vi "Tx Stream Controller (FPGA).vi"() -> ()   [LabVIEW 2016]
doc: "Controls the generation and reception of data transferred from the Host to the FPGA.\nPort 0 receives data from the Port 0 TX Input DMA FIFO and transmits that data to Port 1.\nPort 1 receives data from the Port 1 TX Input DMA FIFO and transmits that data to Port 0."
uses:
  <instrlib>/_niInstr/Streaming/v1/Common/Stream State.ctl
  <vilib>/Platform/TimedLoop/XDataNode/timing_clust.ctl
  <vilib>/Platform/TimedLoop/XDataNode/nitl_modes.ctl
  <vilib>/Platform/TimedLoop/XDataNode/wakeup.ctl
  <instrlib>/_niInstr/CLIP Adapters/v1/FPGA/AXI4-Lite/FXP32 Address - FXP32 Data/Public/CLIP Resources.ctl
  <instrlib>/_niInstr/CLIP Adapters/v1/FPGA/AXI4-Lite/Address Space Collection/niInstr AXI4-Lite Address Space Collection v1 FPGA.lvclass
  C:/Program Files (x86)/National Instruments/LabVIEW 2016/instr.lib/_niInstr/Instruction Framework/v1/FPGA/Interfaces/Address Space Collection/Address Space Collection.lvclass
  <instrlib>/_niInstr/FIFO Register Bus/v1/FPGA/niInstr FIFO Register Bus v1 FPGA.lvclass
  C:/Program Files (x86)/National Instruments/LabVIEW 2016/instr.lib/_niInstr/Instruction Framework/v1/FPGA/Interfaces/Instruction Producer/Instruction Producer.lvclass
  <instrlib>/_niInstr/CLIP Adapters/v1/FPGA/AXI4-Stream/Reader FXP64x1/niInstr AXI4-Stream Reader FXP64x1 v1 FPGA.lvclass
  C:/Program Files (x86)/National Instruments/LabVIEW 2016/instr.lib/_niInstr/CLIP Adapters/v1/FPGA/AXI4-Stream/Reader/niInstr AXI4-Stream Reader v1 FPGA.lvclass
  <instrlib>/_niInstr/CLIP Adapters/v1/FPGA/AXI4-Stream/Writer FXP64x1/niInstr AXI4-Stream Writer FXP64x1 v1 FPGA.lvclass
  C:/Program Files (x86)/National Instruments/LabVIEW 2016/instr.lib/_niInstr/CLIP Adapters/v1/FPGA/AXI4-Stream/Writer/niInstr AXI4-Stream Writer v1 FPGA.lvclass
  <vilib>/rvi/Emulation/niFpgaSctlEmulationGetInTimedLoop.vi
  <vilib>/rvi/Emulation/niFpgaEmulationReportErrorSimple.vi
  <vilib>/rvi/Emulation/niFpgaGetClockAttributes.vi
  <vilib>/rvi/Emulation/niFpgaCriticalErrorInLSC.vi
  <instrlib>/_niInstr/Basic Elements/v1/FPGA/Private/Read U64 FIFO.vi
  <instrlib>/_niInstr/Basic Elements/v1/FPGA/Private/Write U64 FIFO.vi
  <vilib>/rvi/Emulation/niFpgaProcessEmulError.vi
  <vilib>/rvi/eio/common/nirviEmuTemplateMethod_errors.vi
  <vilib>/Platform/TimedLoop/XDataNode/XDataNode.xnode
  <vilib>/eio/EIONode/EIONode.xnode
  <vilib>/Platform/TimedLoop/XDataNode/XDNodeRunTimeDep.lvlib
  <instrlib>/_niInstr/CLIP Adapters/v1/FPGA/AXI4-Stream/Writer/niInstr AXI4-Stream Writer v1 FPGA.lvclass
  <instrlib>/_niInstr/CLIP Adapters/v1/FPGA/AXI4-Stream/Reader/niInstr AXI4-Stream Reader v1 FPGA.lvclass
  <instrlib>/_niInstr/Basic Elements/v1/FPGA/niInstr Basic Elements v1 FPGA.lvlib
  SubVIS/Aurora Stream (NI 6592R) (FPGA).lvlib
  <instrlib>/_niInstr/Streaming/v1/FPGA/niInstr Streaming v1 FPGA.lvlib
  <instrlib>/_niInstr/Streaming/v1/Common/niInstr Streaming v1 Common.lvlib
  <instrlib>/_niInstr/Instruction Framework/v1/FPGA/Top Level Bus/Register Configuration/Register Configuration.lvclass
  <instrlib>/_niInstr/CLIP Adapters/v1/FPGA/AXI4-Lite/FXP32 Address - FXP32 Data/niInstr AXI4-Lite - FXP32 Address - FXP32 Data v1 FPGA.lvclass
panel:
  out "Er.Port 3":u32
  out "Er.Port 2":u32
  out "Er.Port 1":u32
  out "Er.Port 0":u32
  in  "Simulated data":bool
  in  "Reset":bool
  out "Port 3 Link Reset":bool
  out "Port 1 Link Reset":bool
  in  "Port 3 PMA Init":bool
  in  "Port 1 PMA Init":bool
  out "fifo reg bus data 0":u64
  out "fifo reg bus status 0":u32
  in  "fifo reg bus ctrl 0":u32
  in  "Port 0 PMA Init":bool
  in  "Port 2 PMA Init":bool
  out "Port 0 Debug Info":T1
  out "Port 0 Link Reset":bool
  out "Port 2 Link Reset":bool
  out "sFrontEndConfig_Complete":bool
  out "Port 2 Debug Info":T1
  out "stream.state 5":T2
  out "stream.samples transferred 5":u64
  out "stream.metadata 5":u64
  in  "stream.num samples 5":u64
  in  "stream.request state 5":T2
  out "stream.state 4":T2
  out "stream.samples transferred 4":u64
  out "stream.metadata 4":u64
  in  "stream.num samples 4":u64
  in  "stream.request state 4":T2
  in  "stream.request state 0":T2
  in  "stream.num samples 0":u64
  out "stream.metadata 0":u64
  out "stream.samples transferred 0":u64
  out "stream.state 0":T2
  in  "stream.num samples 1":u64
  in  "stream.request state 1":T2
  out "stream.state 1":T2
  out "stream.samples transferred 1":u64
  out "stream.metadata 1":u64
  in  "stream.request state 6":T2
  in  "stream.num samples 6":u64
  out "stream.metadata 6":u64
  out "stream.samples transferred 6":u64
  out "stream.state 6":T2
  in  "stream.request state 7":T2
  in  "stream.num samples 7":u64
  out "stream.metadata 7":u64
  out "stream.samples transferred 7":u64
  out "stream.state 7":T2
  out "Port 3 Debug Info":T1
  in  "stream.request state 2":T2
  in  "stream.num samples 2":u64
  out "stream.metadata 2":u64
  out "stream.samples transferred 2":u64
  out "stream.state 2":T2
  in  "stream.request state 3":T2
  in  "stream.num samples 3":u64
  out "stream.metadata 3":u64
  out "stream.samples transferred 3":u64
  out "stream.state 3":T2
  out "Port 1 Debug Info":T1
  # "Port 0"
  # "Port 2"
  # "Port 1"
  # "Port 3"
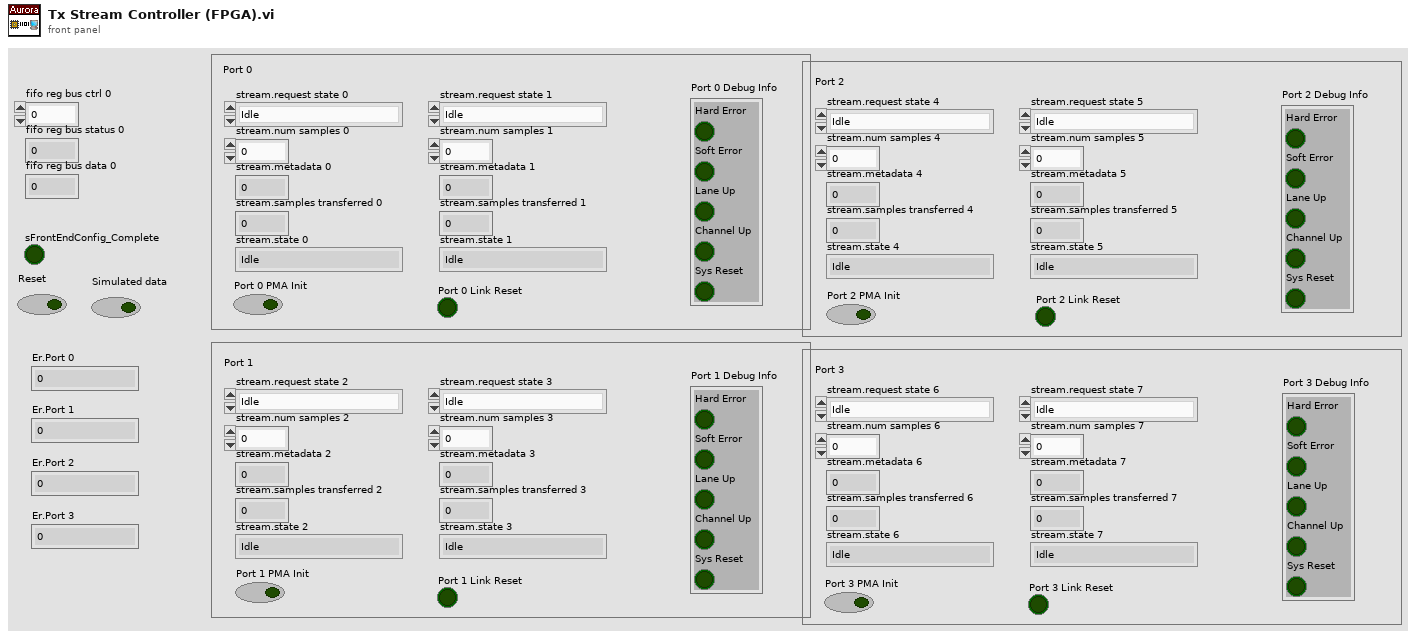
[diagram p1: front panel]
types:
  T1 = cluster{"Hard Error":bool, "Soft Error":bool, "Lane Up":bool, "Channel Up":bool, "Sys Reset":bool}
  T2 = typedef "niInstr Streaming v1 Common.lvlib/Stream State.ctl" = enum8{"Idle", "Finite Transfer", "Continuous", "Done", "Error", "Not Ready", "Cancel"}
  T3 = cluster{"Hard Error":refnum<k21>, "Soft Error":refnum<k21>, "Lane Up":refnum<k21>, "Channel Up":refnum<k21>, "Sys Reset":refnum<k21>}
  T4 = cluster{"m_axis_tvalid":refnum<k21>, "m_axis_tdata":refnum<k21>}
  T5 = cluster{"s_axis_tvalid":refnum<k21>, "s_axis_tdata":refnum<k21>, "s_axis_tready":refnum<k21>}
  T6 = typedef "niInstr AXI4-Lite - FXP32 Address - FXP32 Data v1 FPGA.lvclass/CLIP Resources.ctl" = cluster{"s_axi_araddr":refnum<k21>, "s_axi_arvalid":refnum<k21>, "s_axi_arready":refnum<k21>, "s_axi_rdata":refnum<k21>, "s_axi_rresp":refnum<k21>, "s_axi_rvalid":refnum<k21>, "s_axi_rready":refnum<k21>, "s_axi_awaddr":refnum<k21>, "s_axi_awvalid":refnum<k21>, "s_axi_awready":refnum<k21>, "s_axi_wdata":refnum<k21>, "s_axi_wstrb":refnum<k21>, "s_axi_wvalid":refnum<k21>, "s_axi_wready":refnum<k21>, "s_axi_bresp":refnum<k21>, "s_axi_bvalid":refnum<k21>, "s_axi_bready":refnum<k21>}
  T7 = typedef "XDNodeRunTimeDep.lvlib/timing_clust.ctl" = cluster{"Expected End [f-1]":u64, "Actual End [f-1]":u64, "Finished Late? [f-1]":bool, "Expected End [i-1]":u64, "Actual End [i-1]":u64, "Finished Late? [i-1]":bool, "Expected Start [i]":u64, "Actual Start [i]":u64, "Expected Start [f]":u64, "Actual Start [f]":u64, "Source Name":string, "Structure Name":string, "Period":i64, "Deadline":i64, "Offset":i64, "Start":i64, "Priority":i32, "Timeout":i32, "Mode":T8, "Wakeup Reason":T9, "Error":errorcluster, "Source Type":string, "Secondary Source Type":string, "Global End Time":u64, "Global Start Time":u64, "Frame Duration":u64, "Iteration Duration":u64, "Assigned CPU":i32, "I/O Scan Engine Mode":u32}
  T8 = typedef "XDNodeRunTimeDep.lvlib/nitl_modes.ctl" = enum32{"No Change", "Process missed periods, maintain original phase", "Discard missed periods, maintain original phase", "Process missed periods, ignore original phase", "Discard missed periods, ignore original phase"}
  T9 = typedef "XDNodeRunTimeDep.lvlib/wakeup.ctl" = enum32{"Normal", "Aborted", "Asynchronous wakeup", "Timing source error", "Timed loop error", "Timeout"}
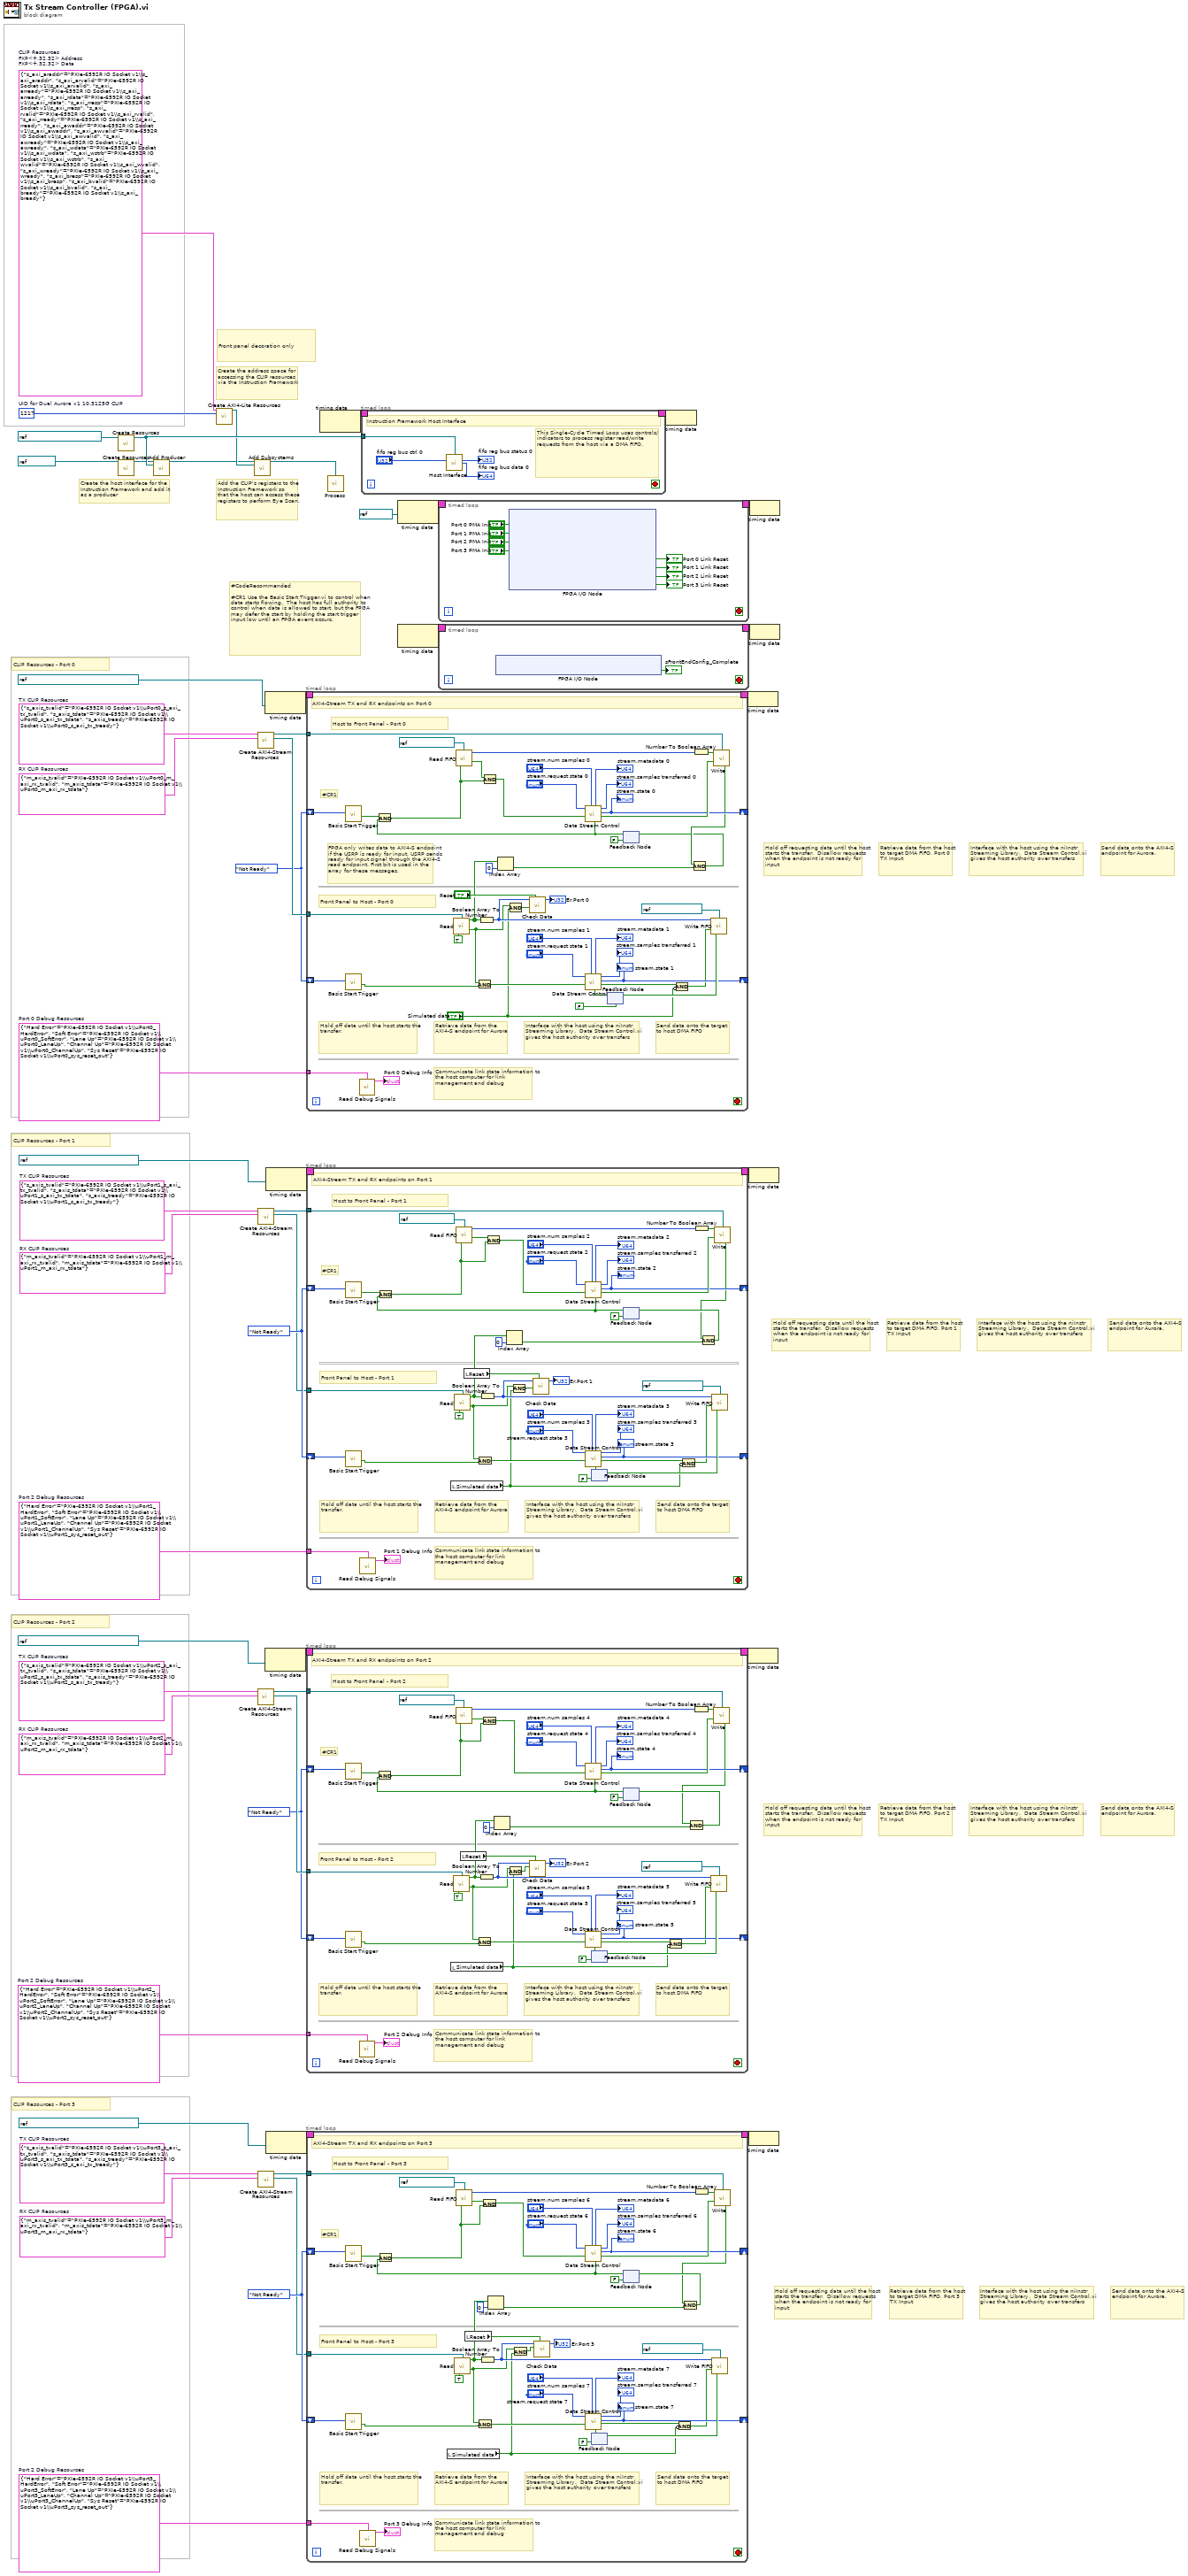
[diagram p0: block diagram]
diagram:
  w10 = T3 {"Hard Error"="PXIe-6592R IO Socket v1\\uPort3_HardError", "Soft Error"="PXIe-6592R IO Socket v1\\uPort3_SoftError", "Lane Up"="PXIe-6592R IO Socket v1\\uPort3_LaneUp", "Channel Up"="PXIe-6592R IO Socket v1\\uPort3_ChannelUp", "Sys Reset"="PXIe-6592R IO Socket v1\\uPort3_sys_reset_out"}  # Port 2 Debug Resources
  w9 = Stream_State."Not Ready" ("stream.state 0")
  w5 = T4 {"m_axis_tvalid"="PXIe-6592R IO Socket v1\\uPort3_m_axi_rx_tvalid", "m_axis_tdata"="PXIe-6592R IO Socket v1\\uPort3_m_axi_rx_tdata"}  # RX CLIP Resources
  w4 = T5 {"s_axis_tvalid"="PXIe-6592R IO Socket v1\\uPort3_s_axi_tx_tvalid", "s_axis_tdata"="PXIe-6592R IO Socket v1\\uPort3_s_axi_tx_tdata", "s_axis_tready"="PXIe-6592R IO Socket v1\\uPort3_s_axi_tx_tready"}  # TX CLIP Resources
  w19 = T3 {"Hard Error"="PXIe-6592R IO Socket v1\\uPort1_HardError", "Soft Error"="PXIe-6592R IO Socket v1\\uPort1_SoftError", "Lane Up"="PXIe-6592R IO Socket v1\\uPort1_LaneUp", "Channel Up"="PXIe-6592R IO Socket v1\\uPort1_ChannelUp", "Sys Reset"="PXIe-6592R IO Socket v1\\uPort1_sys_reset_out"}  # Port 2 Debug Resources
  w18 = Stream_State."Not Ready" ("stream.state 0")
  w14 = T4 {"m_axis_tvalid"="PXIe-6592R IO Socket v1\\uPort1_m_axi_rx_tvalid", "m_axis_tdata"="PXIe-6592R IO Socket v1\\uPort1_m_axi_rx_tdata"}  # RX CLIP Resources
  w13 = T5 {"s_axis_tvalid"="PXIe-6592R IO Socket v1\\uPort1_s_axi_tx_tvalid", "s_axis_tdata"="PXIe-6592R IO Socket v1\\uPort1_s_axi_tx_tdata", "s_axis_tready"="PXIe-6592R IO Socket v1\\uPort1_s_axi_tx_tready"}  # TX CLIP Resources
  w33 = u16 1217  # UID for Dual Aurora x1 10.3125G CLIP
  w34 = T6 {"s_axi_araddr"="PXIe-6592R IO Socket v1\\s_axi_araddr", "s_axi_arvalid"="PXIe-6592R IO Socket v1\\s_axi_arvalid", "s_axi_arready"="PXIe-6592R IO Socket v1\\s_axi_arready", "s_axi_rdata"="PXIe-6592R IO Socket v1\\s_axi_rdata", "s_axi_rresp"="PXIe-6592R IO Socket v1\\s_axi_rresp", "s_axi_rvalid"="PXIe-6592R IO Socket v1\\s_axi_rvalid", "s_axi_rready"="PXIe-6592R IO Socket v1\\s_axi_rready", "s_axi_awaddr"="PXIe-6592R IO Socket v1\\s_axi_awaddr", "s_axi_awvalid"="PXIe-6592R IO Socket v1\\s_axi_awvalid", "s_axi_awready"="PXIe-6592R IO Socket v1\\s_axi_awready", "s_axi_wdata"="PXIe-6592R IO Socket v1\\s_axi_wdata", "s_axi_wstrb"="PXIe-6592R IO Socket v1\\s_axi_wstrb", "s_axi_wvalid"="PXIe-6592R IO Socket v1\\s_axi_wvalid", "s_axi_wready"="PXIe-6592R IO Socket v1\\s_axi_wready", "s_axi_bresp"="PXIe-6592R IO Socket v1\\s_axi_bresp", "s_axi_bvalid"="PXIe-6592R IO Socket v1\\s_axi_bvalid", "s_axi_bready"="PXIe-6592R IO Socket v1\\s_axi_bready"}  # CLIP Resources FXP<+,32,32> Address FXP<+,32,32> Data
  w22 = T3 {"Hard Error"="PXIe-6592R IO Socket v1\\uPort2_HardError", "Soft Error"="PXIe-6592R IO Socket v1\\uPort2_SoftError", "Lane Up"="PXIe-6592R IO Socket v1\\uPort2_LaneUp", "Channel Up"="PXIe-6592R IO Socket v1\\uPort2_ChannelUp", "Sys Reset"="PXIe-6592R IO Socket v1\\uPort2_sys_reset_out"}  # Port 2 Debug Resources
  w40 = T3 {"Hard Error"="PXIe-6592R IO Socket v1\\uPort0_HardError", "Soft Error"="PXIe-6592R IO Socket v1\\uPort0_SoftError", "Lane Up"="PXIe-6592R IO Socket v1\\uPort0_LaneUp", "Channel Up"="PXIe-6592R IO Socket v1\\uPort0_ChannelUp", "Sys Reset"="PXIe-6592R IO Socket v1\\uPort0_sys_reset_out"}  # Port 0 Debug Resources
  w23 = Stream_State."Not Ready" ("stream.state 0")
  w41 = Stream_State."Not Ready" ("stream.state 0")
  w45 = T4 {"m_axis_tvalid"="PXIe-6592R IO Socket v1\\uPort2_m_axi_rx_tvalid", "m_axis_tdata"="PXIe-6592R IO Socket v1\\uPort2_m_axi_rx_tdata"}  # RX CLIP Resources
  w46 = T5 {"s_axis_tvalid"="PXIe-6592R IO Socket v1\\uPort2_s_axi_tx_tvalid", "s_axis_tdata"="PXIe-6592R IO Socket v1\\uPort2_s_axi_tx_tdata", "s_axis_tready"="PXIe-6592R IO Socket v1\\uPort2_s_axi_tx_tready"}  # TX CLIP Resources
  w47 = T4 {"m_axis_tvalid"="PXIe-6592R IO Socket v1\\uPort0_m_axi_rx_tvalid", "m_axis_tdata"="PXIe-6592R IO Socket v1\\uPort0_m_axi_rx_tdata"}  # RX CLIP Resources
  w48 = T5 {"s_axis_tvalid"="PXIe-6592R IO Socket v1\\uPort0_s_axi_tx_tvalid", "s_axis_tdata"="PXIe-6592R IO Socket v1\\uPort0_s_axi_tx_tdata", "s_axis_tready"="PXIe-6592R IO Socket v1\\uPort0_s_axi_tx_tready"}  # TX CLIP Resources
  # "Send data onto the AXI4-S endpoint for Aurora."
  # "Interface with the host using the niInstr Streaming Library.  Data Stream Control.vi gives the host authority over transfers"
  # "Retrieve data from the host to target DMA FIFO, Port 3 TX Input"
  # "Hold off requesting data until the host starts the transfer.  Disallow requests when the endpoint is not ready for input"
  # "Send data onto the AXI4-S endpoint for Aurora."
  # "Interface with the host using the niInstr Streaming Library.  Data Stream Control.vi gives the host authority over transfers"
  # "Retrieve data from the host to target DMA FIFO, Port 2 TX Input"
  # "Hold off requesting data until the host starts the transfer.  Disallow requests when the endpoint is not ready for input"
  # "Send data onto the AXI4-S endpoint for Aurora."
  # "Interface with the host using the niInstr Streaming Library.  Data Stream Control.vi gives the host authority over transfers"
  # "Retrieve data from the host to target DMA FIFO, Port 1 TX Input"
  # "Hold off requesting data until the host starts the transfer.  Disallow requests when the endpoint is not ready for input"
  # "Send data onto the AXI4-S endpoint for Aurora."
  # "Interface with the host using the niInstr Streaming Library.  Data Stream Control.vi gives the host authority over transfers"
  # "Retrieve data from the host to target DMA FIFO, Port 0 TX Input"
  # "Hold off requesting data until the host starts the transfer.  Disallow requests when the endpoint is not ready for input"
  # "CLIP Resources - Port 3"
  # "CLIP Resources - Port 1"
  # "CLIP Resources - Port 2"
  # "CLIP Resources - Port 0"
  # "#CodeRecommended\n\n#CR1 Use the Basic Start Trigger.vi to control when data starts flowing.  The host has full authority to control when data is allowed to start, but the FPGA may defer the start by holding the start trigger input low until an FPGA event occurs."
  # "Add the CLIP's registers to the Instruction Framework so\nthat the host can access these registers to perform Eye Scan."
  # "Create the host interface for the Instruction Framework and add it as a producer"
  # "Create the address space for accessing the CLIP resources via the Instruction Framework"
  # "Front panel decoration only"
  n1 = call <instrlib>:"Create Resources.vi"("instruction fifo"=refnum<k21> "reg.host instruction fifo 0" ("FIFO")) -> ("fifo register bus"=w35:refnum<class "niInstr FIFO Register Bus v1 FPGA.lvclass">)  [unwired: 14 in]
  n2 = call <instrlib>:"Create Resources.vi"("register clock"=refnum<k21> "100MHz" ("Source Name")) -> ("register configuration"=w31:refnum<class "Register Configuration.lvclass">)  [unwired: 14 in]
  n3 = call <instrlib>:"Add Producer.vi"("register configuration in"=w31, "instruction producer"=w35) -> ("register configuration out"=w30:refnum<class "Register Configuration.lvclass">)  [unwired: 13 in]
  n4 = call "Create AXI4-Lite Resources.vi"("CLIP Resources\nFXP<+,32,32> Address\nFXP<+,32,32> Data"=w34, "UID for Dual Aurora x1 10.3125G CLIP"=w33) -> ("niInstr AXI4-Lite Address Space Collection v1 FPGA out"=w32:refnum<class "niInstr AXI4-Lite Address Space Collection v1 FPGA.lvclass">)  [unwired: 13 in]
  n5 = call <instrlib>:"Add Subsystems.vi"("register configuration in"=w30, "subsystems"=w32) -> ("register configuration out"=w29:refnum<class "Register Configuration.lvclass">)  [unwired: 13 in]
  n6 = call "Create AXI4-Stream Resources.vi"("RX CLIP Resources"=w47, "TX CLIP Resources"=w48) -> ("RX niInstr AXI4-Stream Reader FXP64x1 v1 FPGA out"=w42:refnum<class "niInstr AXI4-Stream Reader FXP64x1 v1 FPGA.lvclass">, "TX niInstr AXI4-Stream Reader FXP64x1 v1 FPGA out"=w49:refnum<class "niInstr AXI4-Stream Writer FXP64x1 v1 FPGA.lvclass">)  [unwired: 8 in]
  n7 = call "Create AXI4-Stream Resources.vi"("RX CLIP Resources"=w45, "TX CLIP Resources"=w46) -> ("RX niInstr AXI4-Stream Reader FXP64x1 v1 FPGA out"=w24:refnum<class "niInstr AXI4-Stream Reader FXP64x1 v1 FPGA.lvclass">, "TX niInstr AXI4-Stream Reader FXP64x1 v1 FPGA out"=w25:refnum<class "niInstr AXI4-Stream Writer FXP64x1 v1 FPGA.lvclass">)  [unwired: 8 in]
  n8 = call "Create AXI4-Stream Resources.vi"("RX CLIP Resources"=w14, "TX CLIP Resources"=w13) -> ("RX niInstr AXI4-Stream Reader FXP64x1 v1 FPGA out"=w17:refnum<class "niInstr AXI4-Stream Reader FXP64x1 v1 FPGA.lvclass">, "TX niInstr AXI4-Stream Reader FXP64x1 v1 FPGA out"=w16:refnum<class "niInstr AXI4-Stream Writer FXP64x1 v1 FPGA.lvclass">)  [unwired: 8 in]
  n9 = call "Create AXI4-Stream Resources.vi"("RX CLIP Resources"=w5, "TX CLIP Resources"=w4) -> ("RX niInstr AXI4-Stream Reader FXP64x1 v1 FPGA out"=w8:refnum<class "niInstr AXI4-Stream Reader FXP64x1 v1 FPGA.lvclass">, "TX niInstr AXI4-Stream Reader FXP64x1 v1 FPGA out"=w7:refnum<class "niInstr AXI4-Stream Writer FXP64x1 v1 FPGA.lvclass">)  [unwired: 8 in]
  n10 = node-c288(refnum<k21> "PXIe-6592R IO Socket v1\\Port0_UserClk" ("Source Name")) -> (w52:T7)
  n11 = node-c288(refnum<k21> "PXIe-6592R IO Socket v1\\Port2_UserClk" ("Source Name")) -> (w28:T7)
  n12 = node-c288(refnum<k21> "PXIe-6592R IO Socket v1\\Port1_UserClk" ("Source Name")) -> (w21:T7)
  n13 = node-c288(refnum<k21> "PXIe-6592R IO Socket v1\\Port3_UserClk" ("Source Name")) -> (w12:T7)
  n14 = timed-loop {
    timing: w52 -> [_]
    timing-out: [_] -> w51
    tunnel: w49 -> [w97]
    tunnel: w42 -> [w96]
    shift-right: [w90] -> _
    shift-left: w41 -> [w85]
    shift-right: [w74] -> _
    shift-left: w41 -> [w80]
    tunnel: w40 -> [w72]
    stop <- _ stop-if-true
    # "FPGA only writes data to AXI4-S endpoint if the USRP is ready for input. USRP sends ready for input signal through the AXI4-S read endpoint. First bit is used in the array for these messages."
    # "#CR1"
    # "Communicate link state information to the host computer for link management and debug"
    # "Send data onto the target to host DMA FIFO"
    # "Interface with the host using the niInstr Streaming Library.  Data Stream Control.vi gives the host authority over transfers"
    # "Retrieve data from the AXI4-S endpoint for Aurora"
    # "Hold off data until the host starts the transfer."
    # "Front Panel to Host - Port 0"
    # "Host to Front Panel - Port 0"
    # "AXI4-Stream TX and RX endpoints on Port 0"
    n15 = call <instrlib>:"Basic Start Trigger.vi"("stream.state"=w85) -> ("data valid"=w84:bool)  [unwired: 10 in]
    n16 = call <instrlib>:"Basic Start Trigger.vi"("stream.state"=w80) -> ("data valid"=w79:bool)  [unwired: 10 in]
    n17 = call "Read Debug Signals.vi"("Debug CLIP Resources"=w72) -> ("Debug Info"=→"Port 0 Debug Info":T1)  [unwired: 14 in]
    n18 = call <instrlib>:"Read.vi"("niInstr AXI4-Stream Reader v1 FPGA in"=w96, "ready for output"=TRUE) -> ("tdata"=w60:bool[], "output valid"=w64:bool)  [unwired: 8 in, 4 out]
    n19 = And(x=w64, y=w79) -> (x .and. y?=w73:bool)
    n20 = Boolean Array To Number(Boolean array=w60) -> (number=w67:u64)
    n21 = Index Array(array=w60, index=0) -> (element=w58:bool)
    n22 = Compound Arithmetic op=AND(w64, "Simulated data") -> (w63:bool)
    n23 = call "Check Data.vi"("reset"="Reset", "Input valid"=w63, "IQ Stream"=w67) -> ("errors"=→"Er.Port 0":u32)  [unwired: 8 in]
    n24 = feedback #1(FALSE ("ready for input")) -> (w81:bool)
    n25 = call <instrlib>:"Data Stream Control.vi"("ready for input?"=w81, "stream.num samples 0"="stream.num samples 1", "data valid"=w73, "stream.request state 0"="stream.request state 1") -> ("send data"=w66:bool, "stream.state 0"=w74:T2, "stream.samples transferred 0"=→"stream.samples transferred 1":u64, "stream.metadata 0"=→"stream.metadata 1":u64)  [unwired: 3 in, 1 out]
    "stream.state 1" <- w74
    n26 = feedback #2(FALSE ("ready for input")) -> (w83:bool)
    n27 = And(x=w84, y=w83) -> (x .and. y?=w56:bool)
    n28 = call-poly <instrlib>:"Read FIFO.vi"("fifo"=refnum<k21> "Port 0 TX Input", "ready for output"=w56) -> ("output data"=w92:u64, "output valid"=w57:bool)  [unwired: 12 in]
    n29 = Compound Arithmetic op=AND(w57, w56) -> (w55:bool)
    n30 = call <instrlib>:"Data Stream Control.vi"("ready for input?"=w83, "stream.num samples 0"="stream.num samples 0", "data valid"=w55, "stream.request state 0"="stream.request state 0") -> ("send data"=w91:bool, "stream.state 0"=w90:T2, "stream.samples transferred 0"=→"stream.samples transferred 0":u64, "stream.metadata 0"=→"stream.metadata 0":u64)  [unwired: 3 in, 1 out]
    "stream.state 0" <- w90
    n31 = Compound Arithmetic op=AND(w66, invert "Simulated data") -> (w65:bool)
    n32 = Number To Boolean Array(number=w92) -> (Boolean array=w94:bool[])
    n33 = call-poly <instrlib>:"Write FIFO.vi"("input data"=w67, "fifo"=refnum<k21> "Port 0 RX Output", "input valid"=w65) -> ("ready for input"=w82:bool)  [unwired: 12 in]
    n34 = feedback-in #1(w82) -> ()
    n35 = call <instrlib>:"Write.vi"("tdata"=w94, "niInstr AXI4-Stream Writer v1 FPGA in"=w97, "input valid"=w91) -> ("ready for input"=w54:bool)  [unwired: 12 in]
    n36 = Compound Arithmetic op=AND(w54, w58) -> (w53:bool)
    n37 = feedback-in #2(w53) -> ()
  }
  n38 = timed-loop {
    timing: w28 -> [_]
    timing-out: [_] -> w27
    tunnel: w25 -> [w145]
    tunnel: w24 -> [w144]
    shift-right: [w138] -> _
    shift-left: w23 -> [w133]
    shift-right: [w122] -> _
    shift-left: w23 -> [w128]
    tunnel: w22 -> [w120]
    stop <- _ stop-if-true
    # "#CR1"
    # "Communicate link state information to the host computer for link management and debug"
    # "Send data onto the target to host DMA FIFO"
    # "Interface with the host using the niInstr Streaming Library.  Data Stream Control.vi gives the host authority over transfers"
    # "Retrieve data from the AXI4-S endpoint for Aurora"
    # "Hold off data until the host starts the transfer."
    # "Front Panel to Host - Port 2"
    # "Host to Front Panel - Port 2"
    # "AXI4-Stream TX and RX endpoints on Port 2"
    n39 = call <instrlib>:"Basic Start Trigger.vi"("stream.state"=w133) -> ("data valid"=w132:bool)  [unwired: 10 in]
    n40 = call <instrlib>:"Basic Start Trigger.vi"("stream.state"=w128) -> ("data valid"=w127:bool)  [unwired: 10 in]
    n41 = call "Read Debug Signals.vi"("Debug CLIP Resources"=w120) -> ("Debug Info"=→"Port 2 Debug Info":T1)  [unwired: 14 in]
    n42 = local read "Simulated data"() -> (w110:bool)
    n43 = call <instrlib>:"Read.vi"("niInstr AXI4-Stream Reader v1 FPGA in"=w144, "ready for output"=TRUE) -> ("tdata"=w103:bool[], "output valid"=w113:bool)  [unwired: 8 in, 4 out]
    n44 = local read "Reset"() -> (w115:bool)
    n45 = And(x=w113, y=w127) -> (x .and. y?=w121:bool)
    n46 = Boolean Array To Number(Boolean array=w103) -> (number=w114:u64)
    n47 = Index Array(array=w103, index=0) -> (element=w104:bool)
    n48 = Compound Arithmetic op=AND(w113, w110) -> (w112:bool)
    n49 = call "Check Data.vi"("reset"=w115, "Input valid"=w112, "IQ Stream"=w114) -> ("errors"=→"Er.Port 2":u32)  [unwired: 8 in]
    n50 = feedback #3(FALSE ("ready for input")) -> (w129:bool)
    n51 = call <instrlib>:"Data Stream Control.vi"("ready for input?"=w129, "stream.num samples 0"="stream.num samples 5", "data valid"=w121, "stream.request state 0"="stream.request state 5") -> ("send data"=w111:bool, "stream.state 0"=w122:T2, "stream.samples transferred 0"=→"stream.samples transferred 5":u64, "stream.metadata 0"=→"stream.metadata 5":u64)  [unwired: 3 in, 1 out]
    "stream.state 5" <- w122
    n52 = feedback #4(FALSE ("ready for input")) -> (w131:bool)
    n53 = And(x=w132, y=w131) -> (x .and. y?=w106:bool)
    n54 = call-poly <instrlib>:"Read FIFO.vi"("fifo"=refnum<k21> "Port 2 TX Input", "ready for output"=w106) -> ("output data"=w140:u64, "output valid"=w108:bool)  [unwired: 12 in]
    n55 = And(x=w108, y=w106) -> (x .and. y?=w107:bool)
    n56 = call <instrlib>:"Data Stream Control.vi"("ready for input?"=w131, "stream.num samples 0"="stream.num samples 4", "data valid"=w107, "stream.request state 0"="stream.request state 4") -> ("send data"=w139:bool, "stream.state 0"=w138:T2, "stream.samples transferred 0"=→"stream.samples transferred 4":u64, "stream.metadata 0"=→"stream.metadata 4":u64)  [unwired: 3 in, 1 out]
    "stream.state 4" <- w138
    n57 = Compound Arithmetic op=AND(w111, invert w110) -> (w109:bool)
    n58 = Number To Boolean Array(number=w140) -> (Boolean array=w142:bool[])
    n59 = call-poly <instrlib>:"Write FIFO.vi"("input data"=w114, "fifo"=refnum<k21> "Port 2 RX Output", "input valid"=w109) -> ("ready for input"=w130:bool)  [unwired: 12 in]
    n60 = feedback-in #3(w130) -> ()
    n61 = call <instrlib>:"Write.vi"("tdata"=w142, "niInstr AXI4-Stream Writer v1 FPGA in"=w145, "input valid"=w139) -> ("ready for input"=w101:bool)  [unwired: 12 in]
    n62 = Compound Arithmetic op=AND(w101, w104) -> (w102:bool)
    n63 = feedback-in #4(w102) -> ()
  }
  n64 = timed-loop {
    timing: w21 -> [_]
    timing-out: [_] -> w20
    tunnel: w16 -> [w193]
    tunnel: w17 -> [w192]
    shift-right: [w186] -> _
    shift-left: w18 -> [w181]
    shift-right: [w170] -> _
    shift-left: w18 -> [w176]
    tunnel: w19 -> [w168]
    stop <- _ stop-if-true
    # "#CR1"
    # "Communicate link state information to the host computer for link management and debug"
    # "Send data onto the target to host DMA FIFO"
    # "Interface with the host using the niInstr Streaming Library.  Data Stream Control.vi gives the host authority over transfers"
    # "Retrieve data from the AXI4-S endpoint for Aurora"
    # "Hold off data until the host starts the transfer."
    # "Front Panel to Host - Port 1"
    # "Host to Front Panel - Port 1"
    # "AXI4-Stream TX and RX endpoints on Port 1"
    n65 = call <instrlib>:"Basic Start Trigger.vi"("stream.state"=w181) -> ("data valid"=w180:bool)  [unwired: 10 in]
    n66 = call <instrlib>:"Basic Start Trigger.vi"("stream.state"=w176) -> ("data valid"=w175:bool)  [unwired: 10 in]
    n67 = call "Read Debug Signals.vi"("Debug CLIP Resources"=w168) -> ("Debug Info"=→"Port 1 Debug Info":T1)  [unwired: 14 in]
    n68 = local read "Simulated data"() -> (w157:bool)
    n69 = call <instrlib>:"Read.vi"("niInstr AXI4-Stream Reader v1 FPGA in"=w192, "ready for output"=TRUE) -> ("tdata"=w150:bool[], "output valid"=w160:bool)  [unwired: 8 in, 4 out]
    n70 = local read "Reset"() -> (w162:bool)
    n71 = And(x=w160, y=w175) -> (x .and. y?=w169:bool)
    n72 = Boolean Array To Number(Boolean array=w150) -> (number=w161:u64)
    n73 = Index Array(array=w150, index=0) -> (element=w152:bool)
    n74 = Compound Arithmetic op=AND(w160, w157) -> (w164:bool)
    n75 = call "Check Data.vi"("reset"=w162, "Input valid"=w164, "IQ Stream"=w161) -> ("errors"=→"Er.Port 1":u32)  [unwired: 8 in]
    n76 = feedback #5(FALSE ("ready for input")) -> (w177:bool)
    n77 = call <instrlib>:"Data Stream Control.vi"("ready for input?"=w177, "stream.num samples 0"="stream.num samples 3", "data valid"=w169, "stream.request state 0"="stream.request state 3") -> ("send data"=w159:bool, "stream.state 0"=w170:T2, "stream.samples transferred 0"=→"stream.samples transferred 3":u64, "stream.metadata 0"=→"stream.metadata 3":u64)  [unwired: 3 in, 1 out]
    "stream.state 3" <- w170
    n78 = feedback #6(FALSE ("ready for input")) -> (w179:bool)
    n79 = And(x=w180, y=w179) -> (x .and. y?=w154:bool)
    n80 = call-poly <instrlib>:"Read FIFO.vi"("fifo"=refnum<k21> "Port 1 TX Input", "ready for output"=w154) -> ("output data"=w188:u64, "output valid"=w156:bool)  [unwired: 12 in]
    n81 = And(x=w156, y=w154) -> (x .and. y?=w155:bool)
    n82 = call <instrlib>:"Data Stream Control.vi"("ready for input?"=w179, "stream.num samples 0"="stream.num samples 2", "data valid"=w155, "stream.request state 0"="stream.request state 2") -> ("send data"=w187:bool, "stream.state 0"=w186:T2, "stream.samples transferred 0"=→"stream.samples transferred 2":u64, "stream.metadata 0"=→"stream.metadata 2":u64)  [unwired: 3 in, 1 out]
    "stream.state 2" <- w186
    n83 = Compound Arithmetic op=AND(w159, invert w157) -> (w158:bool)
    n84 = Number To Boolean Array(number=w188) -> (Boolean array=w190:bool[])
    n85 = call-poly <instrlib>:"Write FIFO.vi"("input data"=w161, "fifo"=refnum<k21> "Port 1 RX Output", "input valid"=w158) -> ("ready for input"=w178:bool)  [unwired: 12 in]
    n86 = feedback-in #5(w178) -> ()
    n87 = call <instrlib>:"Write.vi"("tdata"=w190, "niInstr AXI4-Stream Writer v1 FPGA in"=w193, "input valid"=w187) -> ("ready for input"=w149:bool)  [unwired: 12 in]
    n88 = Compound Arithmetic op=AND(w149, w152) -> (w151:bool)
    n89 = feedback-in #6(w151) -> ()
  }
  n90 = timed-loop {
    timing: w12 -> [_]
    timing-out: [_] -> w11
    tunnel: w7 -> [w241]
    tunnel: w8 -> [w240]
    shift-right: [w234] -> _
    shift-left: w9 -> [w229]
    shift-right: [w218] -> _
    shift-left: w9 -> [w224]
    tunnel: w10 -> [w216]
    stop <- _ stop-if-true
    # "#CR1"
    # "Communicate link state information to the host computer for link management and debug"
    # "Send data onto the target to host DMA FIFO"
    # "Interface with the host using the niInstr Streaming Library.  Data Stream Control.vi gives the host authority over transfers"
    # "Retrieve data from the AXI4-S endpoint for Aurora"
    # "Hold off data until the host starts the transfer."
    # "Front Panel to Host - Port 3"
    # "Host to Front Panel - Port 3"
    # "AXI4-Stream TX and RX endpoints on Port 3"
    n91 = call <instrlib>:"Basic Start Trigger.vi"("stream.state"=w229) -> ("data valid"=w228:bool)  [unwired: 10 in]
    n92 = call <instrlib>:"Basic Start Trigger.vi"("stream.state"=w224) -> ("data valid"=w223:bool)  [unwired: 10 in]
    n93 = call "Read Debug Signals.vi"("Debug CLIP Resources"=w216) -> ("Debug Info"=→"Port 3 Debug Info":T1)  [unwired: 14 in]
    n94 = local read "Simulated data"() -> (w206:bool)
    n95 = call <instrlib>:"Read.vi"("niInstr AXI4-Stream Reader v1 FPGA in"=w240, "ready for output"=TRUE) -> ("tdata"=w199:bool[], "output valid"=w209:bool)  [unwired: 8 in, 4 out]
    n96 = local read "Reset"() -> (w211:bool)
    n97 = And(x=w209, y=w223) -> (x .and. y?=w217:bool)
    n98 = Boolean Array To Number(Boolean array=w199) -> (number=w210:u64)
    n99 = Index Array(array=w199, index=0) -> (element=w200:bool)
    n100 = Compound Arithmetic op=AND(w209, w206) -> (w208:bool)
    n101 = call "Check Data.vi"("reset"=w211, "Input valid"=w208, "IQ Stream"=w210) -> ("errors"=→"Er.Port 3":u32)  [unwired: 8 in]
    n102 = feedback #7(FALSE ("ready for input")) -> (w225:bool)
    n103 = call <instrlib>:"Data Stream Control.vi"("ready for input?"=w225, "stream.num samples 0"="stream.num samples 7", "data valid"=w217, "stream.request state 0"="stream.request state 7") -> ("send data"=w207:bool, "stream.state 0"=w218:T2, "stream.samples transferred 0"=→"stream.samples transferred 7":u64, "stream.metadata 0"=→"stream.metadata 7":u64)  [unwired: 3 in, 1 out]
    "stream.state 7" <- w218
    n104 = feedback #8(FALSE ("ready for input")) -> (w227:bool)
    n105 = And(x=w228, y=w227) -> (x .and. y?=w202:bool)
    n106 = call-poly <instrlib>:"Read FIFO.vi"("fifo"=refnum<k21> "Port 3 TX Input", "ready for output"=w202) -> ("output data"=w236:u64, "output valid"=w204:bool)  [unwired: 12 in]
    n107 = And(x=w204, y=w202) -> (x .and. y?=w203:bool)
    n108 = call <instrlib>:"Data Stream Control.vi"("ready for input?"=w227, "stream.num samples 0"="stream.num samples 6", "data valid"=w203, "stream.request state 0"="stream.request state 6") -> ("send data"=w235:bool, "stream.state 0"=w234:T2, "stream.samples transferred 0"=→"stream.samples transferred 6":u64, "stream.metadata 0"=→"stream.metadata 6":u64)  [unwired: 3 in, 1 out]
    "stream.state 6" <- w234
    n109 = Compound Arithmetic op=AND(w207, invert w206) -> (w205:bool)
    n110 = Number To Boolean Array(number=w236) -> (Boolean array=w238:bool[])
    n111 = call-poly <instrlib>:"Write FIFO.vi"("input data"=w210, "fifo"=refnum<k21> "Port 3 RX Output", "input valid"=w205) -> ("ready for input"=w226:bool)  [unwired: 12 in]
    n112 = feedback-in #7(w226) -> ()
    n113 = call <instrlib>:"Write.vi"("tdata"=w238, "niInstr AXI4-Stream Writer v1 FPGA in"=w241, "input valid"=w235) -> ("ready for input"=w197:bool)  [unwired: 12 in]
    n114 = Compound Arithmetic op=AND(w197, w200) -> (w198:bool)
    n115 = feedback-in #8(w198) -> ()
  }
  n116 = node-c288() -> (w39:T7)  [unwired: 1 in]
  n117 = call <instrlib>:"Process.vi"("register configuration"=w29) -> ()  [unwired: 15 in]
  n118 = timed-loop {
    timing: w39 -> [_]
    timing-out: [_] -> w38
    tunnel: w35 -> [w245]
    stop <- _ stop-if-true
    # "This Single-Cycle Timed Loop uses controls/indicators to process register read/write requests from the host via a DMA FIFO."
    # "Instruction Framework Host Interface"
    n119 = call <instrlib>:"Host Interface.vi"("fifo register bus"=w245, "fifo reg bus ctrl 0"="fifo reg bus ctrl 0") -> ("fifo reg bus status 0"=→"fifo reg bus status 0":u32, "fifo reg bus data 0"=→"fifo reg bus data 0":u64)  [unwired: 12 in]
  }
  n120 = node-c288(refnum<k21> "50MHz" ("Source Name")) -> (w44:T7)
  n121 = node-c288() -> (w3:T7)  [unwired: 1 in]
  n122 = timed-loop {
    timing: w44 -> [_]
    timing-out: [_] -> w43
    stop <- _ stop-if-true
    n123 = xnode "FPGA I/O Node"("PXIe-6592R IO Socket v1\\cPort0_PMA_Init"="Port 0 PMA Init", "PXIe-6592R IO Socket v1\\cPort1_PMA_Init"="Port 1 PMA Init", "PXIe-6592R IO Socket v1\\cPort2_PMA_Init"="Port 2 PMA Init", "PXIe-6592R IO Socket v1\\cPort3_PMA_Init"="Port 3 PMA Init") -> ("PXIe-6592R IO Socket v1\\cPort0_link_reset_out"=→"Port 0 Link Reset":bool, "PXIe-6592R IO Socket v1\\cPort1_link_reset_out"=→"Port 1 Link Reset":bool, "PXIe-6592R IO Socket v1\\cPort2_link_reset_out"=→"Port 2 Link Reset":bool, "PXIe-6592R IO Socket v1\\cPort3_link_reset_out"=→"Port 3 Link Reset":bool)  [unwired: 8 in, 8 out]
  }
  n124 = timed-loop {
    timing: w3 -> [_]
    timing-out: [_] -> w2
    stop <- _ stop-if-true
    n125 = xnode "FPGA I/O Node"() -> ("PXIe-6592R IO Socket v1\\sFrontEndConfig_Complete"=→"sFrontEndConfig_Complete":bool)  [unwired: 1 in, 1 out]
  }
  n126 = node-c288(w38) -> ()
  n127 = node-c288(w51) -> ()
  n128 = node-c288(w27) -> ()
  n129 = node-c288(w20) -> ()
  n130 = node-c288(w11) -> ()
  n131 = node-c288(w43) -> ()
  n132 = node-c288(w2) -> ()
